vi "MDAQ_SetCycleDelta.vi"(6 "Delta T (s)":refnum<vi>, 7 "Frequency":refnum<vi>, 8 "error in":errorcluster, 10 "Status_Cluster":T1 {"GATESTOP" format="%04x"; "GATESTRT" format="%04x"; "AMPLITUDE" format="%04x"; "M_CYCLES" format="%04x"; "N_CYCLES" format="%04x"; "STEP" format="%04x"; "BASE" format="%04x"; "CHAN" format="%04x"}, 11 "VISA resource name":refnum<visa-resource-name>) -> (0 "error out":errorcluster, 2 "Status_Cluster Out":T1 {"GATESTOP" format="%04x"; "GATESTRT" format="%04x"; "AMPLITUDE" format="%04x"; "M_CYCLES" format="%04x"; "N_CYCLES" format="%04x"; "STEP" format="%04x"; "BASE" format="%04x"; "CHAN" format="%04x"}, 3 "VISA resource name out":refnum<visa-resource-name>)   [LabVIEW 2021]
uses:
  Status_Cluster.ctl
  CMD_ARG_Enum.ctl
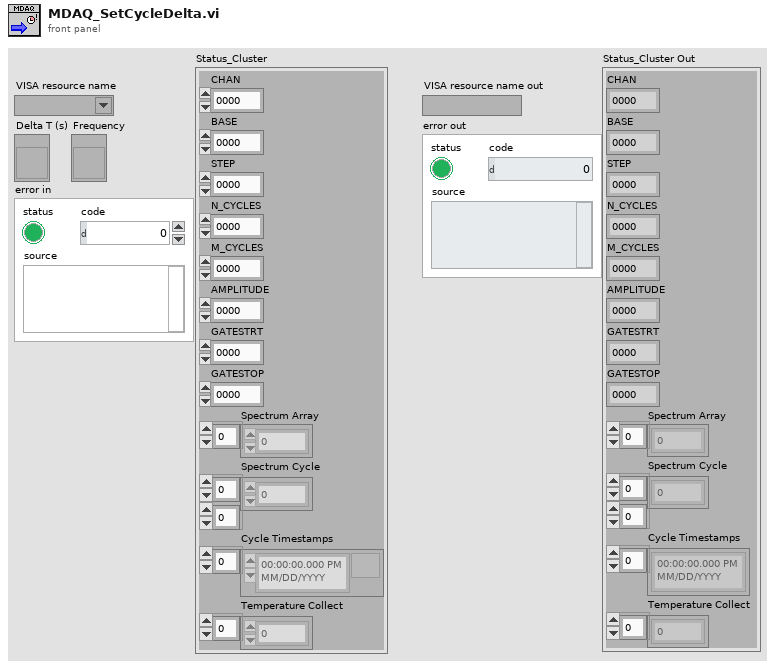
[diagram p1: front panel]
types:
  T1 = typedef "Status_Cluster.ctl" = cluster{"CHAN":u32, "BASE":u32, "STEP":u32, "N_CYCLES":u32, "M_CYCLES":u32, "AMPLITUDE":u32, "GATESTRT":u32, "GATESTOP":u32, "Spectrum Array":u32[], "Spectrum Cycle":u32[][], "Cycle Timestamps":timestamp[], "Temperature Collect":dbl[]}
  T2 = typedef "CMD_ARG_Enum.ctl" = enum16{"N_Cycles", "GateStep", "ASCII_Spectrum", "Waveform", "GateStop", "GateStart", "Amplitude", "Frequency"}
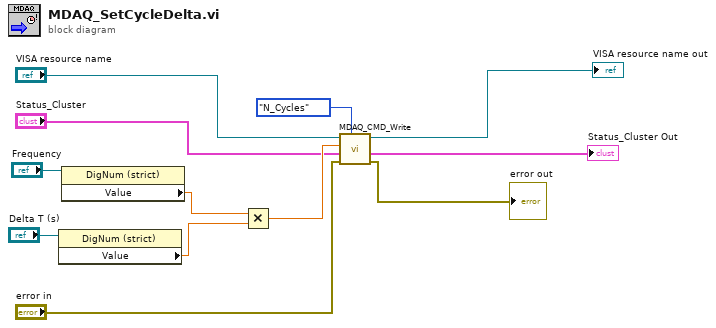
[diagram p0: block diagram]
diagram:
  n1 = property class="DigNum (strict)"(reference="Delta T (s)") -> ("Value"=w7:dbl)  [unwired: 1 in, 2 out]
  n2 = property class="DigNum (strict)"(reference="Frequency") -> ("Value"=w1:dbl)  [unwired: 1 in, 2 out]
  n3 = Multiply(x=w1, y=w7) -> (x*y=w6:dbl)
  n4 = call "MDAQ_CMD_Write.vi"("CMD"=CMD_ARG_Enum."N_Cycles", "error in"="error in", "Status_Cluster"="Status_Cluster", "ARG"=w6, "VISA resource name"="VISA resource name") -> ("error out"=→"error out":errorcluster, "Status_Cluster Out"=→"Status_Cluster Out":T1, "VISA resource name out"=→"VISA resource name out":refnum<visa-resource-name>)  [unwired: 4 in]
